vi "Status check.vi"(8 "error in (no error)":errorcluster, 11 "VISA resource name":refnum<visa-resource-name>) -> (0 "error out":errorcluster, 1 "Target reached?":bool, 2 "Infusing?":bool, 3 "VISA resource name out":refnum<visa-resource-name>, 4 "Stalled?":bool, 5 "Status":string)   [LabVIEW 2016]
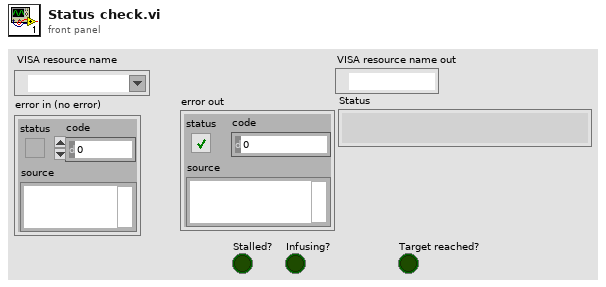
[diagram p1: front panel]
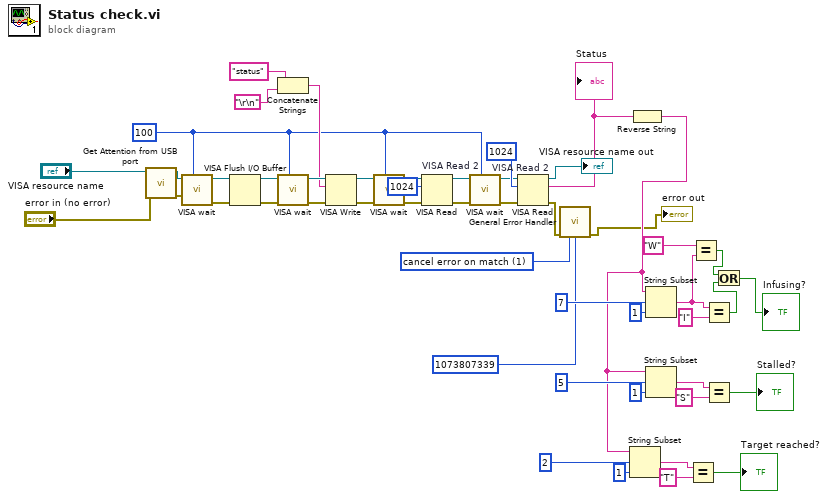
[diagram p0: block diagram]
diagram:
  w10 = 1 items=["no exception", "cancel error on match", "set error on match"] ("[exception action] (none:0)")
  w1 = u32 100 ("milliseconds to wait")
  n1 = call "Get Attention from USB port.vi"("error in (no error)"="error in (no error)", "VISA resource name"="VISA resource name") -> ("error out"=w46:errorcluster, "VISA resource name out"=w47:refnum<visa-resource-name>)  [unwired: 8 in]
  n2 = call <userlib>:"VISA wait.vi"("VISA resource name"=w47, "error in (no error)"=w46, "milliseconds to wait"=w1) -> ("VISA resource name out"=w44:refnum<visa-resource-name>, "error out"=w45:errorcluster)  [unwired: 6 in]
  n3 = VISA Flush I/O Buffer(VISA resource name=w44, error in (no error)=w45) -> (VISA resource name out=w43:refnum<visa-resource-name>, error out=w42:errorcluster)  [unwired: 1 in]
  n4 = Concatenate Strings("status" ("write buffer"), "\r\n") -> (w33:string)
  n5 = call <userlib>:"VISA wait.vi"("VISA resource name"=w43, "error in (no error)"=w42, "milliseconds to wait"=w1) -> ("VISA resource name out"=w40:refnum<visa-resource-name>, "error out"=w41:errorcluster)  [unwired: 6 in]
  n6 = VISA Write(VISA resource name=w40, write buffer=w33, error in (no error)=w41) -> (VISA resource name out=w39:refnum<visa-resource-name>, error out=w38:errorcluster)  [unwired: 1 out]
  n7 = call <userlib>:"VISA wait.vi"("VISA resource name"=w39, "error in (no error)"=w38, "milliseconds to wait"=w1) -> ("VISA resource name out"=w8:refnum<visa-resource-name>, "error out"=w7:errorcluster)  [unwired: 6 in]
  n8 = VISA Read "VISA Read 2"(VISA resource name=w8, byte count=u32 1024, error in (no error)=w7) -> (VISA resource name out=w4:refnum<visa-resource-name>, error out=w5:errorcluster)  [unwired: 2 out]
  n9 = call <userlib>:"VISA wait.vi"("VISA resource name"=w4, "error in (no error)"=w5, "milliseconds to wait"=w1) -> ("VISA resource name out"=w3:refnum<visa-resource-name>, "error out"=w2:errorcluster)  [unwired: 6 in]
  n10 = VISA Read "VISA Read 2"(VISA resource name=w3, byte count=u32 1024, error in (no error)=w2) -> (VISA resource name out=→"VISA resource name out":refnum<visa-resource-name>, read buffer=w32:string, error out=w12:errorcluster)  [unwired: 1 out]
  "Status" <- w32
  n11 = call <vilib>:"General Error Handler.vi"("error in (no error)"=w12, "[exception action] (none:0)"=w10, "[exception code]"=1073807339) -> ("error out"=→"error out":errorcluster)  [unwired: 8 in, 4 out]
  n12 = Reverse String(1:w32) -> (0:w18:string)
  n13 = String Subset(string=w18, offset (0)=2, length (rest)=1 ("length (rest)")) -> (substring=w21:string)
  n14 = String Subset(string=w18, offset (0)=7, length (rest)=1 ("length (rest)")) -> (substring=w14:string)
  n15 = String Subset(string=w18, offset (0)=5, length (rest)=1 ("length (rest)")) -> (substring=w27:string)
  n16 = Equal?(x=w21, y="T") -> (x = y?=→"Target reached?":bool)
  n17 = Equal?(x="W", y=w14) -> (x = y?=w15:bool)
  n18 = Equal?(x=w14, y="I") -> (x = y?=w17:bool)
  n19 = Equal?(x=w27, y="S") -> (x = y?=→"Stalled?":bool)
  n20 = Or(x=w15, y=w17) -> (x .or. y?=→"Infusing?":bool)
